vi "oa_Get Fractional Indices at Specified Time or Speed Positions.vi"(7 "reset? (F)":bool, 9 "position info in":T2, 11 "trigger indices":T1) -> (0 "rpm indices":dbl[](array[numeric]), 1 "position info out":T2, 2 "buffer index":dbl, 3 "fractional indices out":dbl[](array[numeric]), 4 "indices buffer empty?":bool)   [LabVIEW 2017, in "SoundVib_OAUtility.lvlib"]
uses:
  <vilib>/addons/Sound and Vibration/Order Analysis/Utility/SoundVib_OAUtility.lvlib
  <vilib>/addons/Sound and Vibration/Order Analysis/Misc/OAT Position Info.ctl
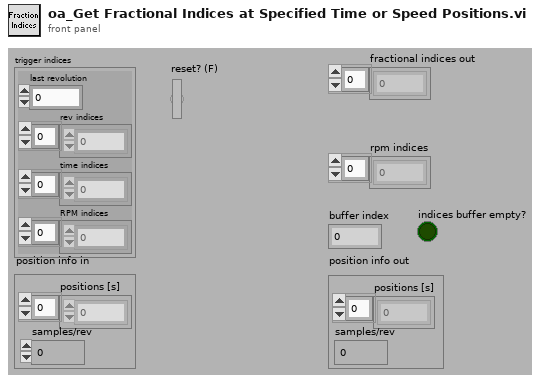
[diagram p1: front panel]
types:
  T1 = cluster{"last revolution":dbl, "rev indices":dbl[], "time indices":dbl[], "RPM indices":dbl[]}
  T2 = typedef "OAT Position Info.ctl" = cluster{"positions [s]":dbl[], "samples/rev":dbl}
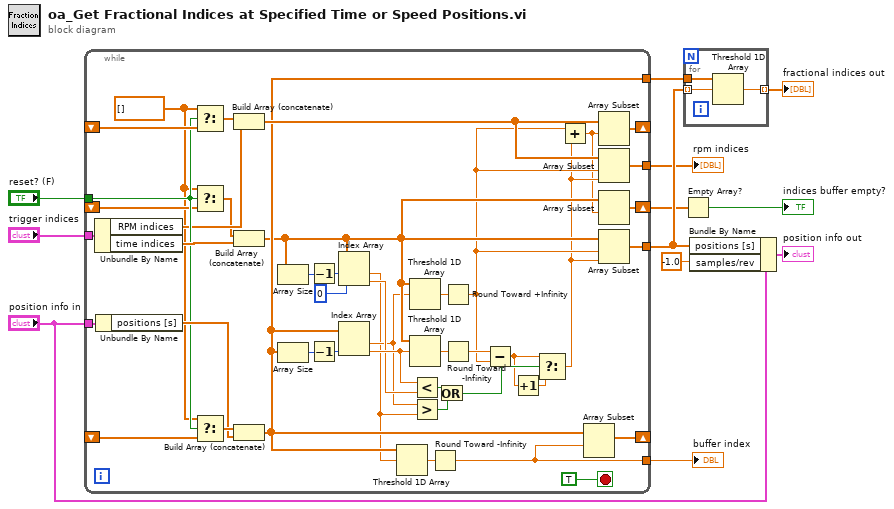
[diagram p0: block diagram]
diagram:
  n1 = while {
    tunnel: "trigger indices" -> [w56]
    tunnel: "position info in" -> [w55]
    tunnel: [w30] -> w10
    tunnel: [w51] -> w9
    shift-right: [w44] -> _
    shift-left: _ -> [w48]
    shift-right: [w40] -> _
    shift-left: _ -> [w49]
    tunnel: "reset? (F)" -> [w39]
    tunnel: [w41] -> w5
    shift-right: [w37] -> w2
    shift-left: _ -> [w38]
    tunnel: [w34] -> w4
    stop <- TRUE stop-if-true
    w29 = dbl[] [] ("positions [s]")
    n2 = Unbundle By Name(w56) -> ("RPM indices"=w36:dbl[], "time indices"=w45:dbl[])
    n3 = Unbundle By Name(w55) -> ("positions [s]"=w46:dbl[])
    n4 = Select(t=w29, s=w39, f=w49) -> (s? t:f=w33:dbl[])
    n5 = Select(t=w29, s=w39, f=w38) -> (s? t:f=w32:dbl[])
    n6 = Select(t=w29, s=w39, f=w48) -> (s? t:f=w47:dbl[])
    n7 = Build Array (concatenate)(w33, w36) -> (w31:dbl[])
    n8 = Build Array (concatenate)(w32, w45) -> (w26:dbl[])
    n9 = Build Array (concatenate)(w47, w46) -> (w30:dbl[])
    n10 = Array Size(array=w26) -> (size(s)=w27:i32)
    n11 = Array Size(array=w30) -> (size(s)=w54:i32)
    n12 = Decrement(x=w27) -> (x-1=w28:i32)
    n13 = Decrement(x=w54) -> (x-1=w53:i32)
    n14 = Index Array(array=w26, index #1=w28, index #2=0 ("index")) -> (element #1=w21:dbl, element #2=w23:dbl)
    n15 = Index Array(array=w30, index #2=w53) -> (element #1=w22:dbl, element #2=w24:dbl)  [unwired: 1 in]
    n16 = Threshold 1D Array(2:w21, 3:w30) -> (0:w43:dbl)  [unwired: 1 in]
    n17 = Threshold 1D Array(2:w22, 3:w26) -> (0:w52:dbl)  [unwired: 1 in]
    n18 = Threshold 1D Array(2:w24, 3:w26) -> (0:w42:dbl)  [unwired: 1 in]
    n19 = Less?(x=w24, y=w23) -> (x < y?=w20:bool)
    n20 = Greater?(x=w22, y=w21) -> (0:w19:bool)
    n21 = Round Toward -Infinity(1:w43) -> (0:w41:dbl)
    n22 = Or(x=w20, y=w19) -> (x .or. y?=w18:bool)
    n23 = Round Toward +Infinity(x=w52) -> (ceil(x): smallest int >= x=w15:dbl)
    n24 = Round Toward -Infinity(1:w42) -> (0:w35:dbl)
    n25 = Subtract(x=w35, y=w15) -> (x-y=w17:dbl)
    n26 = Increment(x=w17) -> (x+1=w16:dbl)
    n27 = Select(t=w17, s=w18, f=w16) -> (s? t:f=w14:dbl)
    n28 = Add(x=w15, y=w14) -> (x+y=w13:dbl)
    n29 = Array Subset(array=w30, index=w41) -> (w44:dbl[])  [unwired: 1 in]
    n30 = Array Subset(array=w31, index=w13) -> (w40:dbl[])  [unwired: 1 in]
    n31 = Array Subset(array=w31, index=w15, length=w14) -> (w34:dbl[])
    n32 = Array Subset(array=w26, index=w13) -> (w37:dbl[])  [unwired: 1 in]
    n33 = Array Subset(array=w26, index=w15, length=w14) -> (w51:dbl[])
  }
  "buffer index" <- w5
  "rpm indices" <- w4
  n34 = Empty Array?(array=w2) -> (empty?=→"indices buffer empty?":bool)
  n35 = for {
    tunnel: w10 -> [w59]
    tunnel: w9 -> [w58] mode=indexing
    tunnel: [w57] -> w8 mode=indexing
    n36 = Threshold 1D Array(2:w58, 3:w59) -> (0:w57:dbl)  [unwired: 1 in]
  }
  "fractional indices out" <- w8
  n37 = Bundle By Name(cluster="position info in", "positions [s]"=w9, "samples/rev"=-1.0) -> (→"position info out":T2)
